vi "send_trigger.vi"(8 "error in (no error)":errorcluster, 10 "trigger":T1, 11 "GenericStage in":refnum<class "GenericStage.lvclass">) -> (0 "error out":errorcluster, 3 "GenericStage out":refnum<class "GenericStage.lvclass">)   [LabVIEW 2010, in "GenericStage.lvclass"]
uses:
  GenericStage.lvclass
  trigger_enum.ctl
  common/classes/GenericToplevelComponent/GenericToplevelComponent/trigger_type_enum.ctl
  common/classes/ErrorController/ErrorController/class_data.vi
  common/classes/ErrorController/ErrorController/ErrorController.lvclass
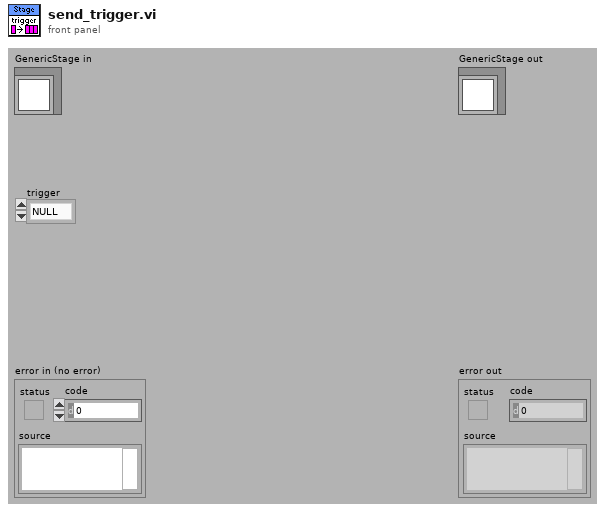
[diagram p1: front panel]
types:
  T1 = typedef "GenericStage.lvclass/trigger_enum.ctl" = enum16{"NULL", "move", "update position", "set origin", "return to origin"}
  T2 = typedef "trigger_type_enum.ctl" = enum8{"external", "internal", "common"}
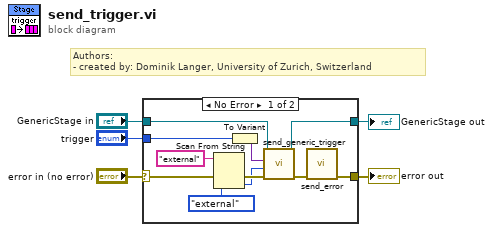
[diagram p0: block diagram]
diagram:
  # "Authors: \n- created by: Dominik Langer, University of Zurich, Switzerland"
  n1 = case shown="No Error" "error in (no error)" {
    selector: "error in (no error)" -> [w9 w18]
    tunnel: [w11 w18] -> w1
    tunnel: [w15 w17] -> w5
    tunnel: "GenericStage in" -> [w14 w17]
    tunnel: "trigger" -> [w16 _]
    frame No Error {
      n2 = Scan From String(input string="external", error in=w9, default 1=trigger_type_enum."external" ("trigger type")) -> (error out=w8:errorcluster, output 1=w7:T2)  [unwired: 2 in, 2 out]
      n3 = To Variant(anything=w16) -> (Variant=w13:variant)
      n4 = call-dynamic "send_generic_trigger.vi"("error in (no error)"=w8, "trigger type"=w7, "trigger variant"=w13, "GenericToplevelComponent in"=w14) -> ("error out"=w12:errorcluster, "GenericToplevelComponent out"=w15:refnum<class "GenericStage.lvclass">)  [unwired: 4 in, 2 out]
      n5 = call "send_error.vi"("error in (no error)"=w12) -> ("error out"=w11:errorcluster)  [unwired: 10 in]
    }
    frame Error {
    }
  }
  "error out" <- w1
  "GenericStage out" <- w5
